vi "SVT Vibration Level (1 Ch).vi"(0 "scaled signal [EU]":waveform(dbl), 1 "integration time [s]":dbl=1.0 format="%.2f", 5 "measurement selection":T1={"RMS"=TRUE, "Running RMS"=FALSE, "Exponential"=FALSE, "Peak"=FALSE, "Max-Min"=FALSE}, 7 "exponential mode":enum16{"Slow", "Fast", "Impulse", "Custom"}(ring)=enum."Fast", 9 "time constant [ms]":dbl=125.0 format="%.2f", 11 "error in (no error)":errorcluster, 12 "restart averaging (F)":bool) -> (3 "exp avg level [EU rms]":waveform(dbl), 4 "RMS level [EU rms]":waveform(dbl), 6 "running RMS level [EU rms]":waveform(dbl), 8 "peak level [EU]":waveform(dbl), 10 "max-min level [EU]":waveform(dbl), 14 "unit label":string, 15 "error out":errorcluster)   [LabVIEW 2017, in "SoundVib_VibrationLevel.lvlib"]
doc: "Computes several vibration level measurements including the root-mean-square (RMS) level, running RMS level, exponential averaged level, peak level, and max-min level. Each instance of this VI maintains its own state; use the N Channel instance of this VI to process an array of channels. This VI operates on time-continuous data; it resets on a discontinuity.<B> Scaled signal [EU]</B> should have a zero DC component. You can attenuate the DC component with hardware AC-coupling filters and with software high-pass filters. Wire data to the <B> scaled signal [EU]</B> input to determine the polymorphic instance to use or manually select the instance."
uses:
  <vilib>/addons/Sound and Vibration/svt_Level/SoundVib_VibrationLevel.lvlib
  <vilib>/addons/Sound and Vibration/svt_Level/SVL Max-Min Level (1 Ch).vi
  <vilib>/addons/Sound and Vibration/svt_Level/SVL Peak Level (1 Ch).vi
  <vilib>/addons/Sound and Vibration/svt_Level/SVL Decimated Exp Avg Level (1 Ch).vi
  <vilib>/addons/Sound and Vibration/svt_Level/SVL Running RMS Level (1 Ch).vi
  <vilib>/addons/Sound and Vibration/svt_Level/SVL RMS Level (1 Ch).vi
  <vilib>/addons/_NISVFA/_Shared subVIs/Common/svc_Engineering Units to Unit Label.vi
  <vilib>/addons/_NISVFA/_Shared subVIs/Common/svc_Unit Label to Engineering Units.vi
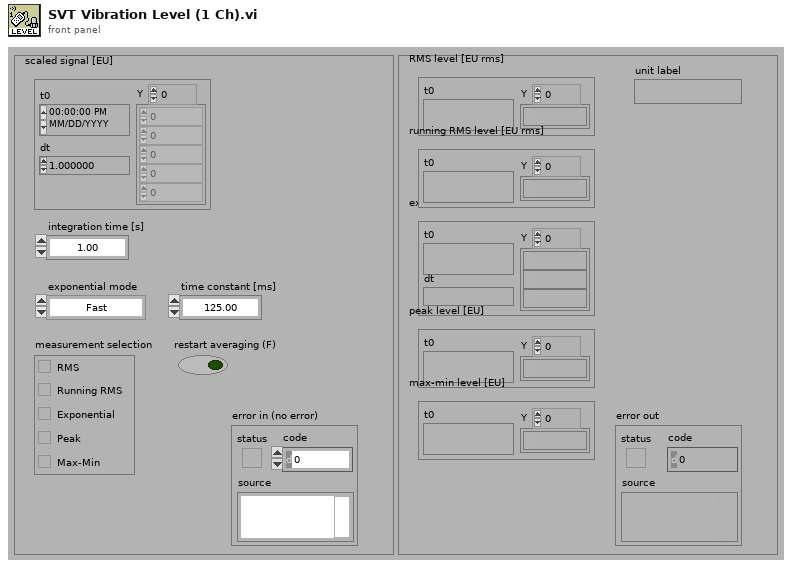
[diagram p1: front panel]
types:
  T1 = cluster{"RMS":bool, "Running RMS":bool, "Exponential":bool, "Peak":bool, "Max-Min":bool}
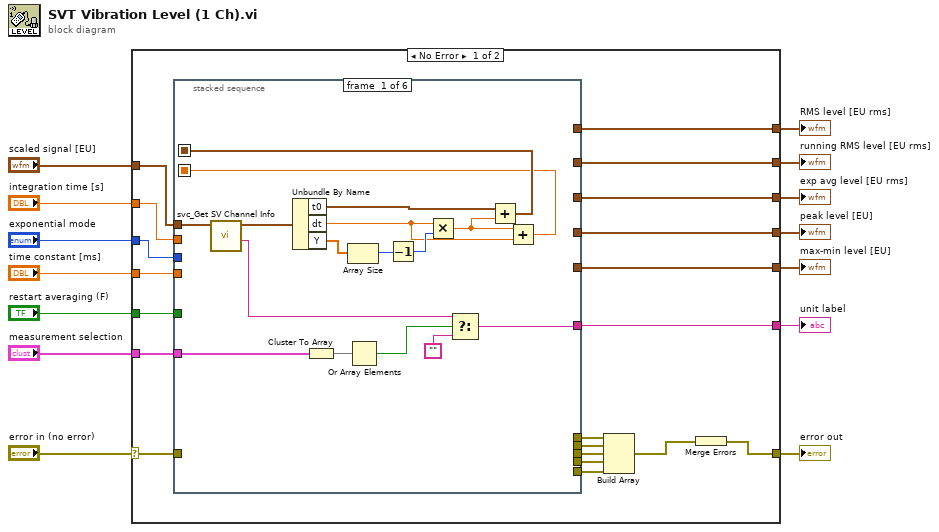
[diagram p0: block diagram]
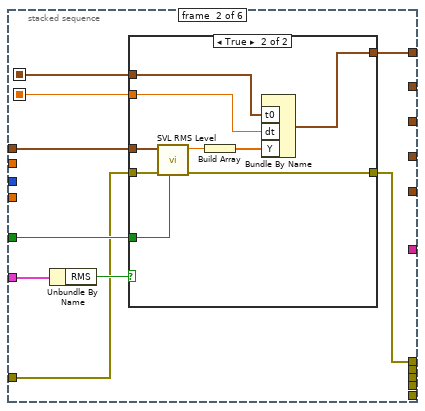
[diagram p2: hidden frame]
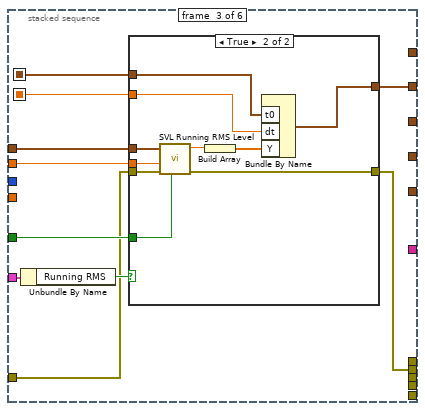
[diagram p4: hidden frame]
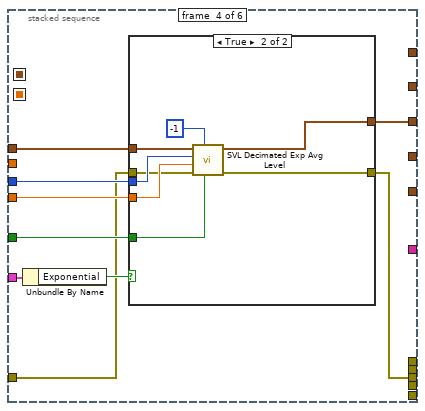
[diagram p6: hidden frame]
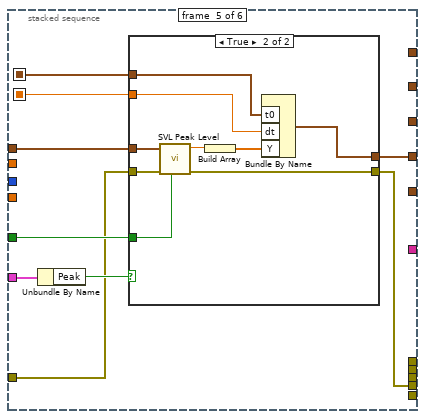
[diagram p8: hidden frame]
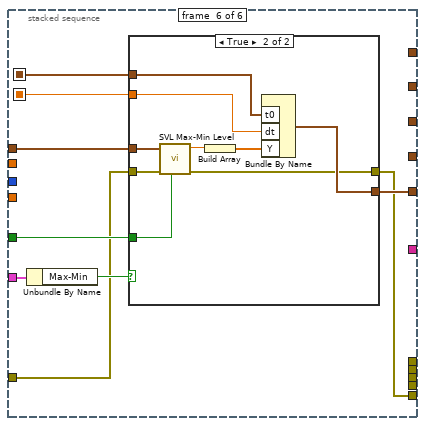
[diagram p10: hidden frame]
diagram:
  n1 = case shown="No Error" "error in (no error)" {
    selector: "error in (no error)" -> [w16 w147]
    tunnel: "scaled signal [EU]" -> [w34 _]
    tunnel: "restart averaging (F)" -> [w33 _]
    tunnel: [w32 _] -> w12
    tunnel: [w31 _] -> w11
    tunnel: "integration time [s]" -> [w30 _]
    tunnel: "exponential mode" -> [w29 _]
    tunnel: "time constant [ms]" -> [w28 _]
    tunnel: [w27 _] -> w7
    tunnel: [w26 _] -> w6
    tunnel: [w25 _] -> w5
    tunnel: "measurement selection" -> [w24 _]
    tunnel: [w15 _] -> w3
    tunnel: [w17 w147] -> w2
    frame No Error {
      n2 = stacked-sequence {
        seq-local: [w43 _ _ _ _ _] -> [_ w54 w74 _ w112 w131]
        seq-local: [w46 _ _ _ _ _] -> [_ w55 w75 _ w113 w132]
        tunnel: w24 -> [w40 w59 w79 w99 w117 w136]
        tunnel: w34 -> [w42 w57 w77 w97 w115 w134]
        tunnel: w33 -> [_ w56 w76 w96 w114 w133]
        tunnel: [_ w53 _ _ _ _] -> w32
        tunnel: [_ _ w73 _ _ _] -> w31
        tunnel: w30 -> [_ _ w72 _ _ _]
        tunnel: w29 -> [_ _ _ w95 _ _]
        tunnel: w28 -> [_ _ _ w94 _ _]
        tunnel: [_ _ _ w93 _ _] -> w27
        tunnel: [_ _ _ _ w111 _] -> w26
        tunnel: [_ _ _ _ _ w130] -> w25
        tunnel: w16 -> [_ w52 w71 w92 w110 w129]
        tunnel: [_ w51 _ _ _ _] -> w23
        tunnel: [_ _ w70 _ _ _] -> w22
        tunnel: [_ _ _ w91 _ _] -> w21
        tunnel: [_ _ _ _ w109 _] -> w20
        tunnel: [_ _ _ _ _ w128] -> w19
        tunnel: [w39 _ _ _ _ _] -> w15
        frame #0 {
          n3 = call <vilib>:"svc_Get SV Channel Info.vi"("scaled signal [EU]"=w42) -> ("unit label"=w35:string, "dup scaled signal [EU]"=w41:waveform(dbl))  [unwired: 5 in, 4 out]
          n4 = Unbundle By Name(w41) -> ("t0"=w48:timestamp, "dt"=w44:dbl, "Y"=w50:dbl[])
          n5 = Cluster To Array(cluster=w40) -> (array=w38:bool[])
          n6 = Array Size(array=w50) -> (size(s)=w49:i32)
          n7 = Or Array Elements(Boolean array=w38) -> (logical OR=w37:bool)
          n8 = Decrement(x=w49) -> (x-1=w47:i32)
          n9 = Multiply(x=w44, y=w47) -> (x*y=w45:dbl)
          n10 = Select(t=w35, s=w37, f="") -> (s? t:f=w39:string)
          n11 = Add(x=w48, y=w45) -> (x+y=w46:timestamp)
          n12 = Add(x=w45, y=w44) -> (x+y=w43:dbl)
        }
        frame #1 {
          n13 = Unbundle By Name(w59) -> ("RMS"=w58:bool)
          n14 = case shown="True" w58 {
            tunnel: w57 -> [_ w69]
            tunnel: w56 -> [_ w68]
            tunnel: w55 -> [_ w65]
            tunnel: w54 -> [_ w64]
            tunnel: [_ w63] -> w53
            tunnel: w52 -> [w60 w62]
            tunnel: [w60 w61] -> w51
            frame False {
            }
            frame True {
              n15 = call-poly <vilib>:"SVL RMS Level.vi"("restart averaging (F)"=w68, "error in (no error)"=w62, "scaled signal [EU]"=w69) -> ("error out"=w61:errorcluster, "RMS level [EU rms]"=w67:dbl)  [unwired: 6 in, 1 out]
              n16 = Build Array(w67) -> (w66:dbl[])
              n17 = Bundle By Name("t0"=w65, "dt"=w64, "Y"=w66) -> (w63:waveform(dbl))  [unwired: 1 in]
            }
          }
        }
        frame #2 {
          n18 = Unbundle By Name(w79) -> ("Running RMS"=w78:bool)
          n19 = case shown="True" w78 {
            tunnel: w77 -> [_ w87]
            tunnel: w76 -> [_ w86]
            tunnel: w75 -> [_ w89]
            tunnel: w74 -> [_ w88]
            tunnel: [_ w84] -> w73
            tunnel: w72 -> [_ w83]
            tunnel: w71 -> [w80 w82]
            tunnel: [w80 w81] -> w70
            frame False {
            }
            frame True {
              n20 = call-poly <vilib>:"SVL Running RMS Level.vi"("restart averaging (F)"=w86, "error in (no error)"=w82, "integration time [s]"=w83, "scaled signal [EU]"=w87) -> ("error out"=w81:errorcluster, "running RMS level [EU rms]"=w85:dbl)  [unwired: 4 in, 2 out]
              n21 = Build Array(w85) -> (w90:dbl[])
              n22 = Bundle By Name("t0"=w89, "dt"=w88, "Y"=w90) -> (w84:waveform(dbl))  [unwired: 1 in]
            }
          }
        }
        frame #3 {
          n23 = Unbundle By Name(w99) -> ("Exponential"=w98:bool)
          n24 = case shown="True" w98 {
            tunnel: w97 -> [_ w108]
            tunnel: w96 -> [_ w107]
            tunnel: w95 -> [_ w106]
            tunnel: w94 -> [_ w105]
            tunnel: [_ w103] -> w93
            tunnel: w92 -> [w100 w102]
            tunnel: [w100 w101] -> w91
            frame False {
            }
            frame True {
              n25 = call-poly <vilib>:"SVL Decimated Exp Avg Level.vi"("restart averaging (F)"=w107, "decimation factor"=-1, "error in (no error)"=w102, "time constant [ms]"=w105, "exponential mode"=w106, "scaled signal [EU]"=w108) -> ("error out"=w101:errorcluster, "decimated exp avg level [EU rms]"=w103:waveform(dbl))  [unwired: 1 in, 3 out]
            }
          }
        }
        frame #4 {
          n26 = Unbundle By Name(w117) -> ("Peak"=w116:bool)
          n27 = case shown="True" w116 {
            tunnel: w115 -> [_ w124]
            tunnel: w114 -> [_ w123]
            tunnel: w113 -> [_ w126]
            tunnel: w112 -> [_ w125]
            tunnel: [_ w121] -> w111
            tunnel: w110 -> [w118 w120]
            tunnel: [w118 w119] -> w109
            frame False {
            }
            frame True {
              n28 = call-poly <vilib>:"SVL Peak Level.vi"("restart averaging (F)"=w123, "error in (no error)"=w120, "scaled signal [EU]"=w124) -> ("error out"=w119:errorcluster, "peak level [EU]"=w122:dbl)  [unwired: 6 in, 1 out]
              n29 = Build Array(w122) -> (w127:dbl[])
              n30 = Bundle By Name("t0"=w126, "dt"=w125, "Y"=w127) -> (w121:waveform(dbl))  [unwired: 1 in]
            }
          }
        }
        frame #5 {
          n31 = Unbundle By Name(w136) -> ("Max-Min"=w135:bool)
          n32 = case shown="True" w135 {
            tunnel: w134 -> [_ w143]
            tunnel: w133 -> [_ w142]
            tunnel: w132 -> [_ w145]
            tunnel: w131 -> [_ w144]
            tunnel: [_ w140] -> w130
            tunnel: w129 -> [w137 w139]
            tunnel: [w137 w138] -> w128
            frame False {
            }
            frame True {
              n33 = call-poly <vilib>:"SVL Max-Min Level.vi"("restart averaging (F)"=w142, "error in (no error)"=w139, "scaled signal [EU]"=w143) -> ("error out"=w138:errorcluster, "max-min level [EU]"=w141:dbl)  [unwired: 4 in, 3 out]
              n34 = Build Array(w141) -> (w146:dbl[])
              n35 = Bundle By Name("t0"=w145, "dt"=w144, "Y"=w146) -> (w140:waveform(dbl))  [unwired: 1 in]
            }
          }
        }
      }
      n36 = Build Array(w23, w22, w21, w20, w19) -> (w18:errorcluster[])
      n37 = Merge Errors(w18) -> (w17:errorcluster)
    }
    frame Error {
    }
  }
  "error out" <- w2
  "exp avg level [EU rms]" <- w7
  "RMS level [EU rms]" <- w12
  "running RMS level [EU rms]" <- w11
  "peak level [EU]" <- w6
  "max-min level [EU]" <- w5
  "unit label" <- w3
